vi "Handle Picture Shortcut Activation.vi"(8 "MenuRef":refnum<k9>, 9 "Container State":T1, 10 "state in":T3={"Draw Options"={"Text Color"=16777238, "Wing Color"=16751616, "Dial Outline Color"=13816530, "Sky Color"=3381759, "Ground Color"=8213043, "Horizon Line Color"=16777225, "Outline Color"=0, "Dial Background Color"=5987163, "Draw Wings"=TRUE, "Draw Text"=TRUE, "Font Name"="Helvetica", "Angle units"=enum."Radians"}} caption="State", 11 "data in":T2) -> ()   [LabVIEW 2017, in "Attitude Indicator.xctl"]
uses:
  <vilib>/robotics/Controls/Attitude Indicator/Attitude Indicator.xctl
  <vilib>/robotics/Controls/Attitude Indicator/_Attitude Indicator Support Files/Attitude Indicator State.ctl
  <vilib>/robotics/Controls/Attitude Indicator/Attitude Picture/Draw Options.ctl
  <vilib>/robotics/Controls/Utilities/Angle Units.ctl
  <vilib>/robotics/Controls/Attitude Indicator/_Attitude Indicator Support Files/Attitude Indicator Data.ctl
  <vilib>/_xctls/Container State.ctl
  <vilib>/robotics/Controls/Utilities/NI_Robotics_Control Utilities.lvlib
  <vilib>/robotics/Controls/Attitude Indicator/Attitude Picture/NI_Robotics_Attitude Picture.lvlib
  <vilib>/_xctls/XControlSupport.lvlib
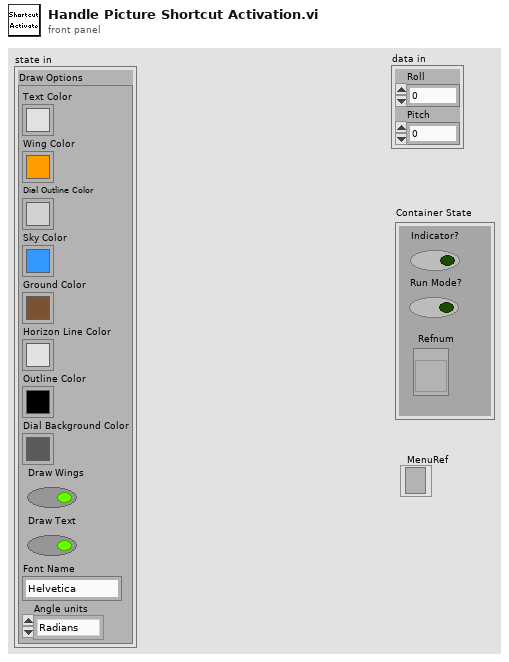
[diagram p1: front panel]
types:
  T1 = typedef "XControlSupport.lvlib/Container State.ctl" = cluster{"Indicator?":bool, "Run Mode?":bool, " Refnum":refnum<vi>}
  T2 = typedef "Attitude Indicator.xctl/Attitude Indicator Data.ctl" = cluster{"Roll":dbl, "Pitch":dbl}
  T3 = typedef "Attitude Indicator.xctl/Attitude Indicator State.ctl" = cluster{"Draw Options":T4}
  T4 = typedef "NI_Robotics_Attitude Picture.lvlib/Draw Options.ctl" = cluster{"Text Color":u32, "Wing Color":u32, "Dial Outline Color":u32, "Sky Color":u32, "Ground Color":u32, "Horizon Line Color":u32, "Outline Color":u32, "Dial Background Color":u32, "Draw Wings":bool, "Draw Text":bool, "Font Name":string, "Angle units":T5}
  T5 = typedef "NI_Robotics_Control Utilities.lvlib/Angle Units.ctl" = enum16{"Radians", "Degrees"}
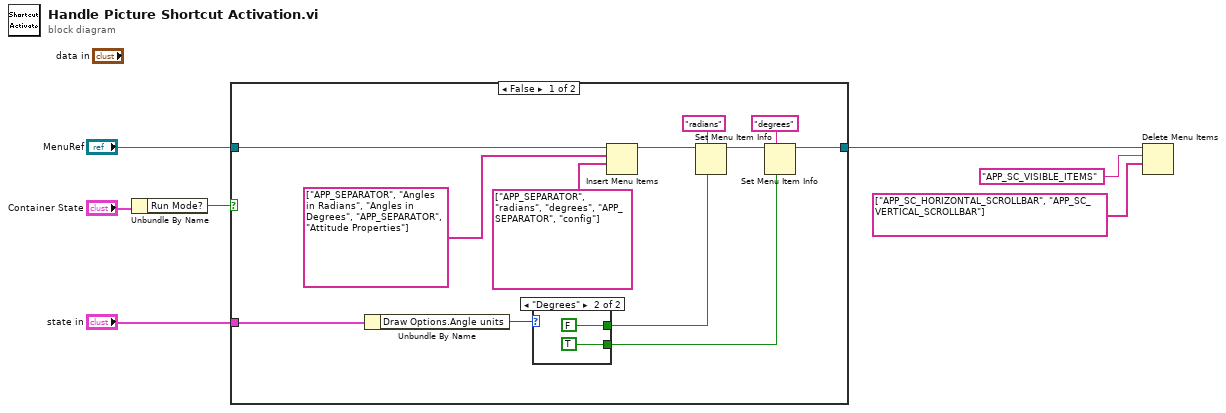
[diagram p0: block diagram]
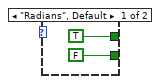
[diagram p2: hidden frame]
diagram:
  n1 = Unbundle By Name("Container State") -> ("Run Mode?"=w6:bool)
  n2 = case shown="False" w6 {
    tunnel: "MenuRef" -> [w10 w24]
    tunnel: "state in" -> [w9 _]
    tunnel: [w8 w24] -> w1
    frame False {
      n3 = Unbundle By Name(w9) -> ("Draw Options.Angle units"=w17:T5)
      n4 = case shown="\"Degrees\"" w17 {
        tunnel: [TRUE FALSE] -> w18
        tunnel: [FALSE TRUE] -> w19
        frame "Radians", Default {
        }
        frame "Degrees" {
        }
      }
      n5 = Insert Menu Items(7:string[] ["APP_SEPARATOR", "radians", "degrees", "APP_SEPARATOR", "config"], 8:string[] ["APP_SEPARATOR", "Angles in Radians", "Angles in Degrees", "APP_SEPARATOR", "Attitude Properties"], 9:w10) -> (3:w14:refnum<k9>)  [unwired: 3 in, 2 out]
      n6 = Set Menu Item Info(6:w18, 7:"radians" ("item tag"), 11:w14) -> (3:w13:refnum<k9>)  [unwired: 4 in, 1 out]
      n7 = Set Menu Item Info(6:w19, 7:"degrees" ("item tag"), 11:w13) -> (3:w8:refnum<k9>)  [unwired: 4 in, 1 out]
    }
    frame True {
    }
  }
  n8 = Delete Menu Items(7:string[] ["APP_SC_HORIZONTAL_SCROLLBAR", "APP_SC_VERTICAL_SCROLLBAR"], 8:"APP_SC_VISIBLE_ITEMS", 9:w1) -> ()  [unwired: 1 in, 2 out]
